vi "Write to Buffer.vi"(8 "error in (no error)":errorcluster, 10 "Data":string, 11 "Terminal in":refnum<class "Terminal.lvclass">) -> (0 "error out":errorcluster, 3 "Terminal out":refnum<class "Terminal.lvclass">)   [LabVIEW 2020, in "Terminal.lvlib" / "Terminal.lvclass"]
uses:
  Terminal.lvclass
  Terminal.lvclass/Terminal.ctl
  TermBuffer/TermBuffer.lvclass
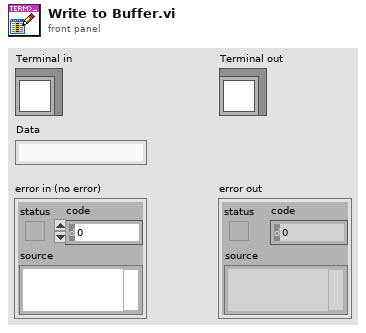
[diagram p1: front panel]
types:
  T1 = typedef "Terminal.lvlib/Terminal.lvclass/Buffers.ctl" = cluster{"Scrollback":refnum<class "TermBuffer.lvclass">, "Primary":refnum<class "TermBuffer.lvclass">, "Alternate":refnum<class "TermBuffer.lvclass">}
  T2 = typedef "Terminal.lvlib/Terminal.lvclass/Ref Data.ctl" = cluster{"Connection":refnum<class "Connection.lvclass">, "Read Loop Running":bool, "Parse State":T3, "Terminal Options":T9, "Font Metrics":T12, "Scroll":i32, "Close Read Loop":bool, "Buffer":T8, "Pause Read Loop":bool}
  T3 = typedef "Terminal.lvlib/Terminal.lvclass/Parse State.ctl" = cluster{"Buffer State":T4, "Cursor":T5, "Attributes":T7, "Active Buffer":T8}
  T4 = typedef "Terminal.lvlib/Terminal.lvclass/Buffer State.ctl" = cluster{"Sequence":string, "ESC":bool, "Alt Buf":bool}
  T5 = typedef "Terminal.lvlib/Terminal.lvclass/Cursor.ctl" = cluster{"Cur":T6, "Saved":T6}
  T6 = typedef "Terminal.lvlib/Terminal.lvclass/Position.ctl" = cluster{"Row":i32, "Col":i32}
  T7 = typedef "Terminal.lvlib/Text Attributes.ctl" = cluster{"FG":u32, "BG":u32, "Bold":bool, "Italic":bool, "Underline":bool, "Strike":bool, "Inverse":bool}
  T8 = typedef "Terminal.lvlib/Buffer.ctl" = enum16{"Primary", "Alternate"}
  T9 = typedef "Terminal.lvlib/Terminal Options.ctl" = cluster{"Implied CR with LF":bool, "Local Echo":bool, "Tab Width":i32, "Color Scheme":T10, "Default FG":T11, "Default BG":T11, "History Length":i32, "Font Face":string, "Font Size":i16, "Rows":i32, "Cols":i32}
  T10 = typedef "Terminal.lvlib/Color Scheme.ctl" = cluster{"Black":u32, "Red":u32, "Green":u32, "Yellow":u32, "Blue":u32, "Magenta":u32, "Cyan":u32, "White":u32, "Bright Black":u32, "Bright Red":u32, "Bright Green":u32, "Bright Yellow":u32, "Bright Blue":u32, "Bright Magenta":u32, "Bright Cyan":u32, "Bright White":u32}
  T11 = typedef "Terminal.lvlib/Color.ctl" = i8
  T12 = typedef "Terminal.lvlib/Terminal.lvclass/Font Metrics.ctl" = cluster{"Width":i16, "Height":i16}
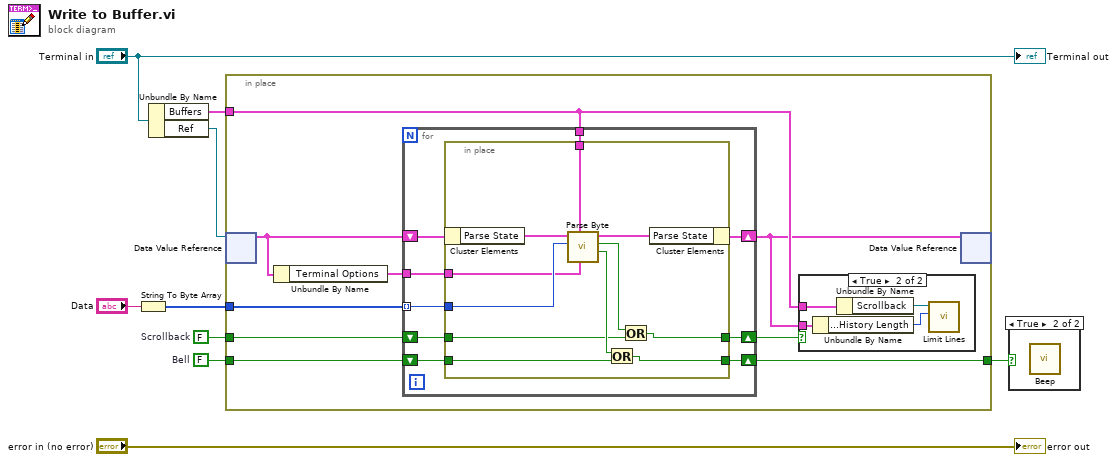
[diagram p0: block diagram]
diagram:
  w1 = FALSE  # Scrollback
  w4 = FALSE  # Bell
  n1 = String To Byte Array(string="Data") -> (unsigned byte array=w5:u8[])
  n2 = Unbundle By Name("Terminal in") -> ("Buffers"=w2:T1, "Ref"=w7:refnum<data-value>)
  n3 = in-place {
    in-place-border: w5 -> [w18]
    in-place-border: w4 -> [w17]
    in-place-border: [w16] -> w3
    in-place-border: w2 -> [w11]
    in-place-border: w1 -> [w13]
    n4 = in-place-dvr #1(w7) -> (w15:T2)  [unwired: 1 out]
    n5 = Unbundle By Name(w15) -> ("Terminal Options"=w14:T9)
    n6 = for {
      tunnel: w18 -> [w29] mode=indexing
      shift-right: [w30] -> w10
      shift-left: w15 -> [w31]
      shift-right: [w27] -> w16
      shift-left: w17 -> [w28]
      tunnel: w14 -> [w26]
      tunnel: w11 -> [w25]
      shift-right: [w23] -> w12
      shift-left: w13 -> [w24]
      n7 = in-place {
        in-place-border: w29 -> [w42]
        in-place-border: w28 -> [w40]
        in-place-border: [w39] -> w27
        in-place-border: w26 -> [w38]
        in-place-border: w25 -> [w37]
        in-place-border: w24 -> [w35]
        in-place-border: [w33] -> w23
        n8 = in-place-cluster #2(w31) -> ("Parse State"=w32:T3)
        n9 = call "Parse Byte.vi"("Terminal Options"=w38, "Buffers"=w37, "Byte"=w42, "Parse State In"=w32) -> ("Bell"=w36:bool, "Scrollback"=w34:bool, "Parse State"=w41:T3)  [unwired: 5 in]
        n10 = Or(x=w36, y=w40) -> (x .or. y?=w39:bool)
        n11 = Or(x=w34, y=w35) -> (x .or. y?=w33:bool)
        n12 = in-place-cluster #2("Parse State"=w41) -> (w30:T2)
      }
    }
    n13 = case shown="True" w12 {
      tunnel: w11 -> [_ w22]
      tunnel: w10 -> [_ w21]
      frame False {
      }
      frame True {
        n14 = Unbundle By Name(w21) -> ("Terminal Options.History Length"=w19:i32)
        n15 = Unbundle By Name(w22) -> ("Scrollback"=w20:refnum<class "TermBuffer.lvclass">)
        n16 = call "Limit Lines.vi"("Count"=w19, "TermBuffer in"=w20) -> ()  [unwired: 8 in, 2 out]
      }
    }
    n17 = in-place-dvr #1(w10) -> ()  [unwired: 2 out]
  }
  n18 = case shown="True" w3 {
    frame False {
    }
    frame True {
      n19 = call <vilib>:"Beep.vi"() -> ()  [unwired: 12 in]
    }
  }
  "error out" <- "error in (no error)"
  "Terminal out" <- "Terminal in"
